vi "Parse Signed Response.vi"(8 "error in (no error)":errorcluster, 11 "body in":string) -> (0 "error out":errorcluster, 2 "signed result cluster":T1, 3 "body out":string)   [LabVIEW 2014, in "Random JSON API.lvlib"]
uses:
  Random JSON API.lvlib
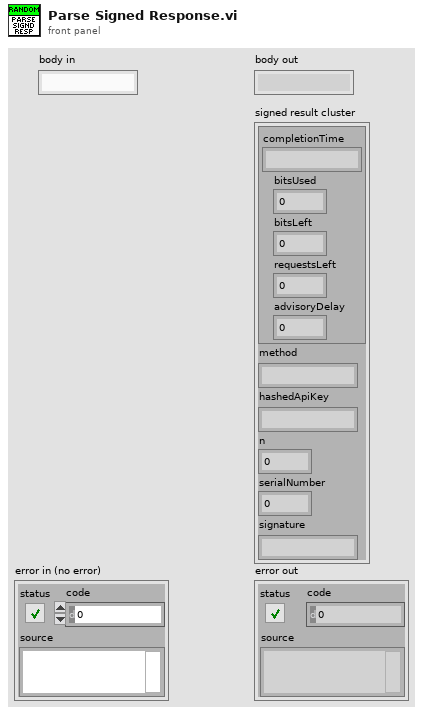
[diagram p1: front panel]
types:
  T1 = cluster{"result cluster":cluster{"completionTime":string, "bitsUsed":i32, "bitsLeft":i32, "requestsLeft":i32, "advisoryDelay":i32}, "method":string, "hashedApiKey":string, "n":i32, "serialNumber":i32, "signature":string}
  T2 = cluster{"completionTime":string, "bitsUsed":i32, "bitsLeft":i32, "requestsLeft":i32, "advisoryDelay":i32}
  T3 = cluster{"result cluster":cluster{"completionTime":string, "bitsUsed":i32, "bitsLeft":i32, "requestsLeft":i32, "advisoryDelay":i32}, string, string, i32, i32, string}
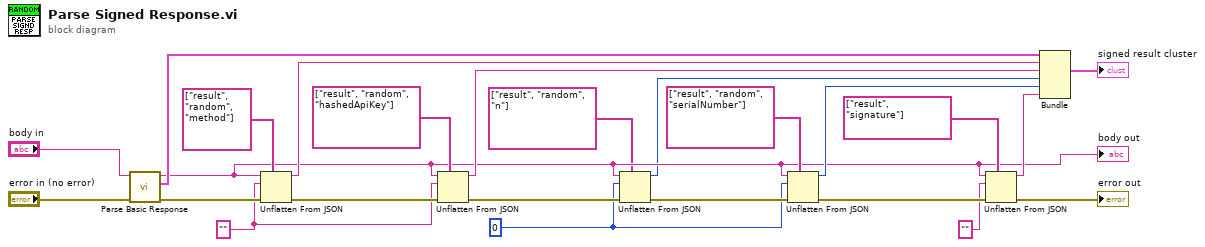
[diagram p0: block diagram]
diagram:
  w5 = 0
  w1 = ""
  n1 = call "Parse Basic Response.vi"("error in (no error)"="error in (no error)", "body in"="body in") -> ("error out"=w23:errorcluster, "result cluster"=w21:T2, "body out"=w4:string)  [unwired: 7 in]
  "body out" <- w4
  n2 = Unflatten From JSON(path=string[] ["result", "random", "method"], JSON string=w4, type and defaults=w1, error in (no error)=w23) -> (value=w18:string, error out=w17:errorcluster)  [unwired: 3 in]
  n3 = Unflatten From JSON(path=string[] ["result", "random", "hashedApiKey"], JSON string=w4, type and defaults=w1, error in (no error)=w17) -> (value=w16:string, error out=w7:errorcluster)  [unwired: 3 in]
  n4 = Unflatten From JSON(path=string[] ["result", "random", "n"], JSON string=w4, type and defaults=w5, error in (no error)=w7) -> (value=w2:i32, error out=w6:errorcluster)  [unwired: 3 in]
  n5 = Unflatten From JSON(path=string[] ["result", "random", "serialNumber"], JSON string=w4, type and defaults=w5, error in (no error)=w6) -> (value=w12:i32, error out=w11:errorcluster)  [unwired: 3 in]
  n6 = Unflatten From JSON(path=string[] ["result", "signature"], JSON string=w4, type and defaults="", error in (no error)=w11) -> (value=w8:string, error out=→"error out":errorcluster)  [unwired: 3 in]
  n7 = Bundle("result cluster"=w21, w18, w16, w2, w12, w8) -> (→"signed result cluster":T3)  [unwired: 1 in]
